vi "MeasureBreakdown.vi"(1 "Microsites":refnum<k24>, 2 "Junction Name":string, 7 ".NET Refnum":refnum<k24>, 9 "Function":string, 12 "appended path":path, 13 "new file path (Not A Path if cancelled)":path, 14 "UiDefinition":T1) -> (15 "error out":errorcluster)   [LabVIEW 2020]
uses:
  UIReferences.ctl
  C:/Users/User/Desktop/Automation/CurrentVersion/LabviewDXFViewer/bin/Release/LabviewDXFViewer.exe
  LabviewDXFViewer/bin/Release/LabviewDXFViewer.exe
  <vilib>/Utility/file.llb/Write Delimited Spreadsheet (string).vi
  <vilib>/Utility/file.llb/Write Delimited Spreadsheet (DBL).vi
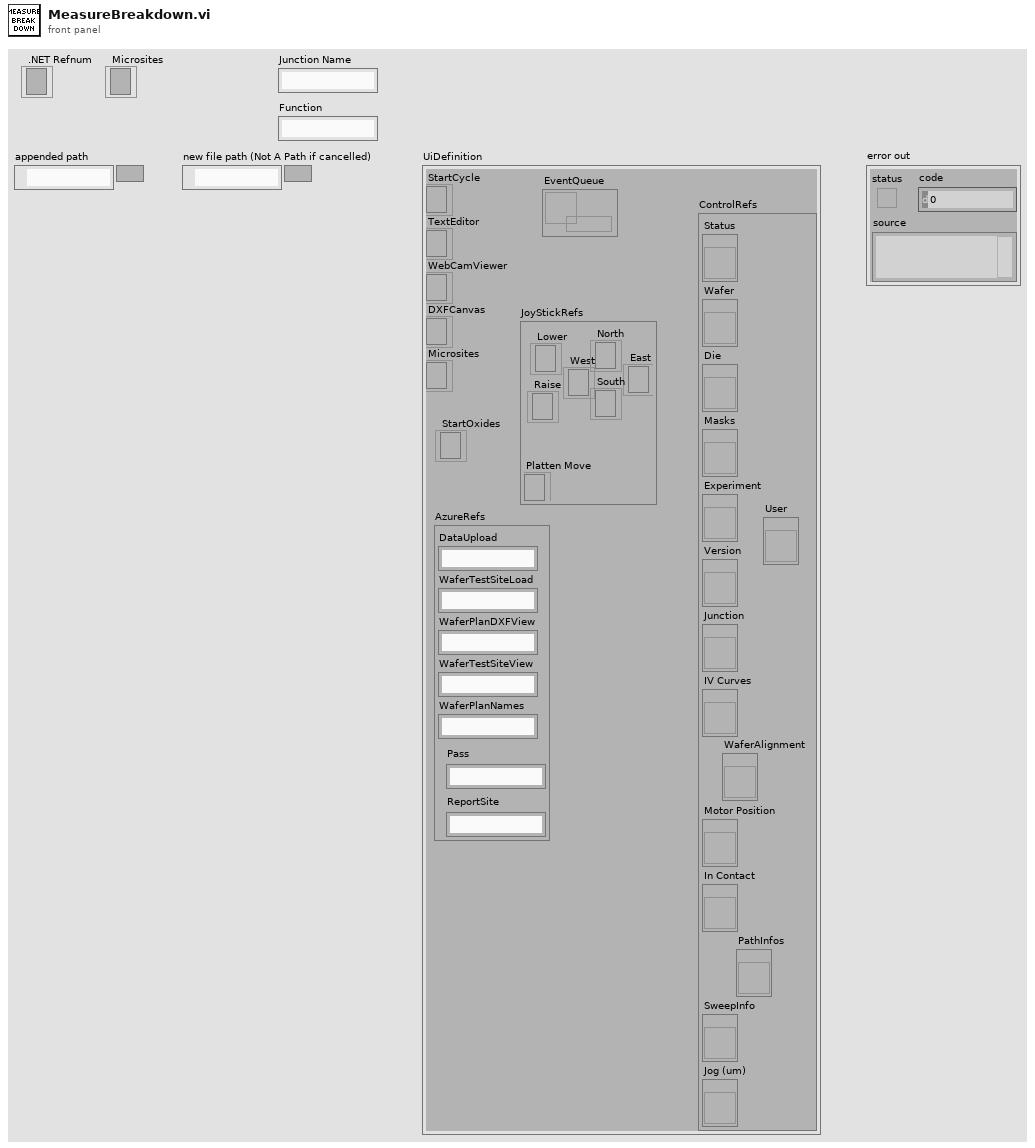
[diagram p1: front panel]
types:
  T1 = typedef "UIReferences.ctl" = cluster{"StartCycle":refnum<k24>, "TextEditor":refnum<k24>, "WebCamViewer":refnum<k24>, "DXFCanvas":refnum<k24>, "Microsites":refnum<k24>, "JoyStickRefs":cluster{"North":refnum<k24>, "Lower":refnum<k24>, "Raise":refnum<k24>, "Platten Move":refnum<k24>, "West":refnum<k24>, "East":refnum<k24>, "South":refnum<k24>}, "AzureRefs":cluster{"DataUpload":string, "WaferTestSiteLoad":string, "WaferPlanDXFView":string, "WaferTestSiteView":string, "WaferPlanNames":string, "Pass":string, "ReportSite":string}, "ControlRefs":cluster{"Status":refnum<vi>, "Wafer":refnum<vi>, "Die":refnum<vi>, "Masks":refnum<vi>, "Experiment":refnum<vi>, "Version":refnum<vi>, "Junction":refnum<vi>, "IV Curves":refnum<vi>, "Motor Position":refnum<vi>, "In Contact":refnum<vi>, "SweepInfo":refnum<vi>, "Jog (um)":refnum<vi>, "PathInfos":refnum<vi>, "User":refnum<vi>, "WaferAlignment":refnum<vi>}, "EventQueue":refnum<queue>, "StartOxides":refnum<k24>}
  T2 = typedef "CapacitanceInfos.ctl" = cluster{"Conductance":dbl, "CapacitanceIV":dbl, "Intercept":dbl, "CapacitanceSW":dbl, "Sum":dbl, "CapacitanceInfos":T3[], "CapacitancePhase":dbl, "dC/dV":dbl}
  T3 = typedef "CapacitanceRecord.ctl" = cluster{"Freq":dbl, "Vpp":dbl, "PhaseS":dbl, "Irms":dbl, "PhaseC":dbl, "Theta":dbl, "VDrive":dbl, "Capacitance":dbl, "Other":dbl}
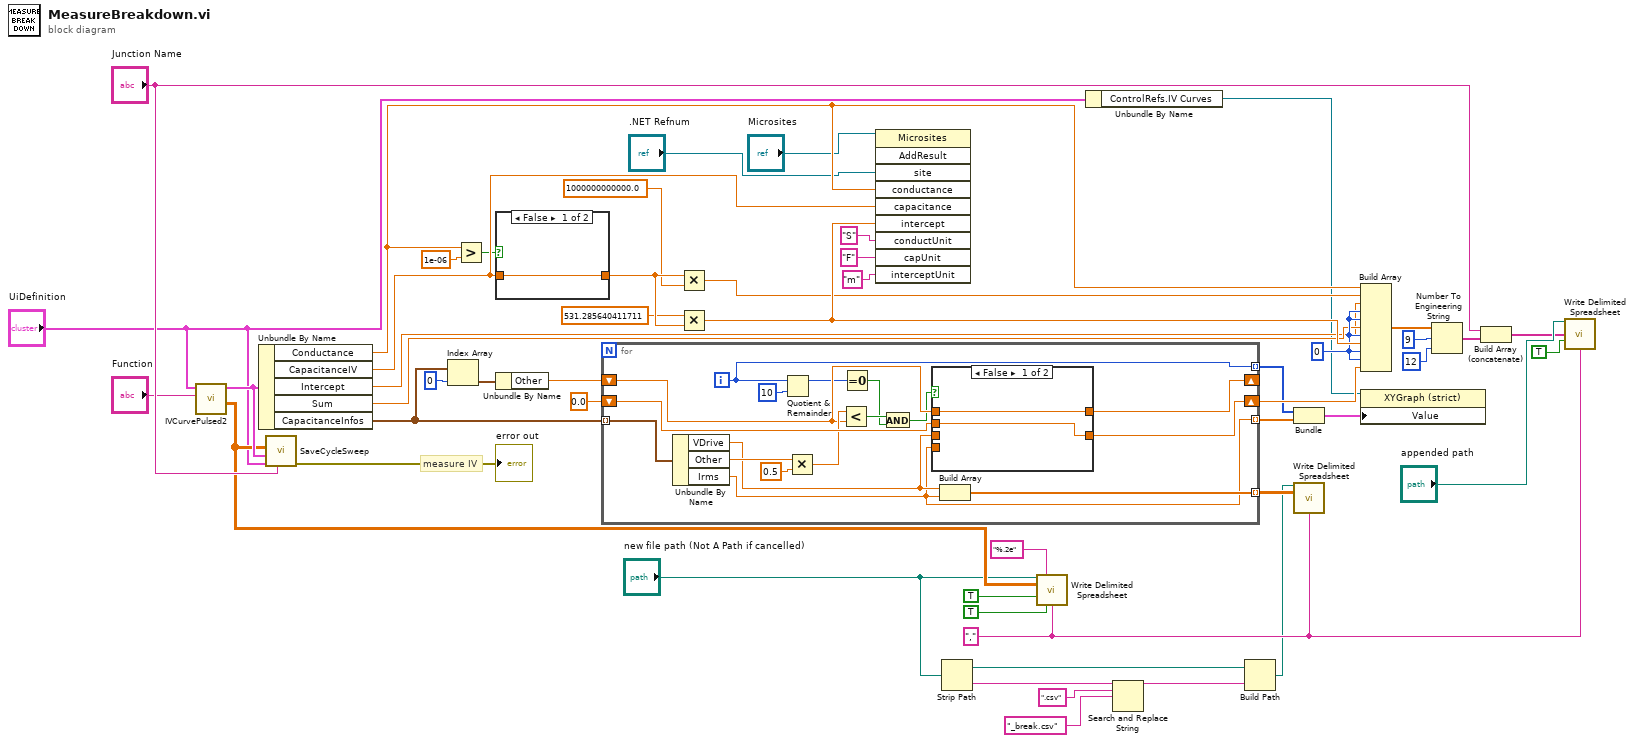
[diagram p0: block diagram]
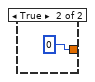
[diagram p3: hidden frame]
diagram:
  w11 = "," ("delimiter (\\t)")
  w41 = 0
  # "measure IV"
  n1 = call "IVCurvePulsed2.vi"("Program"="Function", "UiDefinition"="UiDefinition") -> ("appended array"=w20:dbl[][], "InfoCluster"=w33:T2)  [unwired: 8 in]
  n2 = Unbundle By Name(w33) -> ("Conductance"=w40:dbl, "CapacitanceIV"=w39:dbl, "Intercept"=w23:dbl, "Sum"=w24:dbl, "CapacitanceInfos"=w44:T3[])
  n3 = call "SaveCycleSweep.vi"("JunctionName"="Junction Name", "UiDefinition 2"="UiDefinition", "InfoCluster"=w33, "appended array"=w20) -> ("error out"=→"error out":errorcluster)  [unwired: 7 in]
  n4 = Index Array(array=w44, index=0) -> (element=w46:T3)
  n5 = Greater?(x=w40, y=1e-06) -> (0:w27:bool)
  n6 = case shown="False" w27 {
    tunnel: [w53 0] -> w51
    tunnel: w39 -> [w53 _]
    frame False {
    }
    frame True {
    }
  }
  n7 = Unbundle By Name(w46) -> ("Other"=w47:dbl)
  n8 = for {
    tunnel: w44 -> [w71] mode=indexing
    tunnel: [w59] -> w42 mode=indexing
    tunnel: [w60] -> w43 mode=indexing
    shift-right: [w64] -> _
    shift-left: w47 -> [w65]
    shift-right: [w69] -> w48
    shift-left: 0.0 ("Vpp") -> [w68]
    tunnel: [w61] -> w13 mode=indexing
    i -> [w59]
    n9 = Unbundle By Name(w71) -> ("VDrive"=w62:dbl, "Other"=w63:dbl, "Irms"=w60:dbl)
    n10 = Quotient & Remainder(x=w59, y=10) -> (x-y*floor(x/y)=w55:i32)  [unwired: 1 out]
    n11 = Multiply(x=w63, y=0.5) -> (x*y=w67:dbl)
    n12 = Less?(x=w67, y=w65) -> (x < y?=w70:bool)
    n13 = Equal To 0?(x=w55) -> (x = 0?=w56:bool)
    n14 = And(x=w70, y=w56) -> (x .and. y?=w57:bool)
    n15 = case shown="False" w57 {
      tunnel: w62 -> [_ w75]
      tunnel: [w73 w75] -> w69
      tunnel: w68 -> [w73 _]
      tunnel: [w72 w74] -> w64
      tunnel: w65 -> [w72 _]
      tunnel: w60 -> [_ w74]
      frame False {
      }
      frame True {
      }
    }
    n16 = Build Array(w62, w60) -> (w61:dbl[])
  }
  n17 = Multiply(x=w51, y=1000000000000.0) -> (x*y=w25:dbl)
  n18 = Multiply(x=531.285640411711, y=w51) -> (x*y=w52:dbl)
  n19 = invoke class="Microsites" method="AddResult"(reference="Microsites", "site"=".NET Refnum", "conductance"=w40, "capacitance"=w39, "intercept"=w52, "conductUnit"="S", "capUnit"="F", "interceptUnit"="m") -> ()  [unwired: 2 in, 10 out]
  n20 = Strip Path(path="new file path (Not A Path if cancelled)") -> (stripped path=w5:path, name=w9:string)
  n21 = call-poly <vilib>:"Write Delimited Spreadsheet.vi"("file path (dialog if empty)"="new file path (Not A Path if cancelled)", "format (%.3f)"="%.2e", "2D data"=w20, "append to file? (new file:F)"=TRUE, "transpose? (no:F)"=TRUE, "delimiter (\\t)"=w11) -> ()  [unwired: 8 in, 2 out]
  n22 = Unbundle By Name("UiDefinition") -> ("ControlRefs.IV Curves"=w2:refnum<vi>)
  n23 = Search and Replace String(input string=w9, search string=".csv", replace string="_break.csv" ("replace string (\"\")")) -> (result string=w6:string)  [unwired: 5 in, 3 out]
  n24 = Build Path(base path=w5, name or relative path=w6) -> (appended path=w4:path)
  n25 = Bundle(w42, w43) -> (w1:cluster{i32[], dbl[]})  [unwired: 1 in]
  n26 = call-poly <vilib>:"Write Delimited Spreadsheet.vi"("file path (dialog if empty)"=w4, "2D data"=w13, "delimiter (\\t)"=w11) -> ()  [unwired: 11 in, 2 out]
  n27 = Build Array(w40, w25, w23, w41, w41, w24, w41, w52, w41, w41, w48) -> (w22:dbl[])
  n28 = property class="XYGraph (strict)"(reference=w2, "Value"=w1) -> ()  [unwired: 1 in, 2 out]
  n29 = Number To Engineering String(2:i16 12 ("precision (6)"), 3:i16 9 ("width (-)"), 4:w22) -> (0:w14:string[])  [unwired: 1 in]
  n30 = Build Array (concatenate)("Junction Name", w14) -> (w16:string[])
  n31 = call-poly <vilib>:"Write Delimited Spreadsheet.vi"("file path (dialog if empty)"="appended path", "1D data"=w16, "append to file? (new file:F)"=TRUE, "delimiter (\\t)"=w11) -> ()  [unwired: 10 in, 2 out]
